vi "Cast IOLink Data.vi"(11 "System State In":map{string, dbl}(c390)) -> (3 "System State Out":map{string, dbl}(c390))   [LabVIEW 2024, in "Hardware Controller.lvlib"]
uses:
  Hardware Controller.lvlib
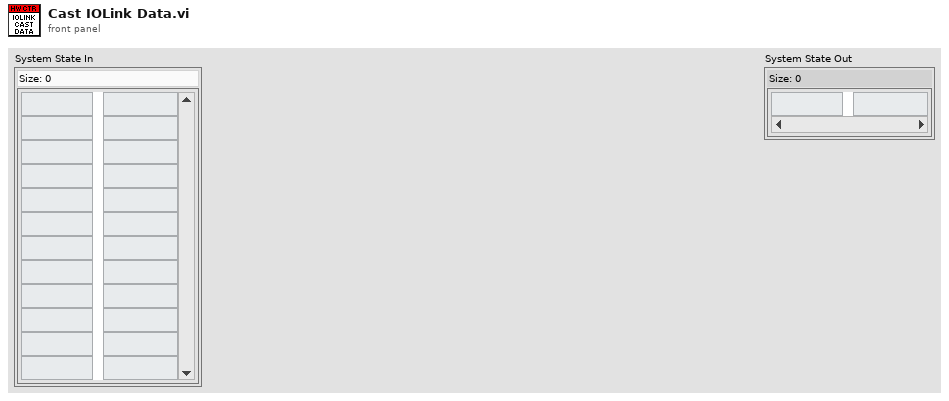
[diagram p1: front panel]
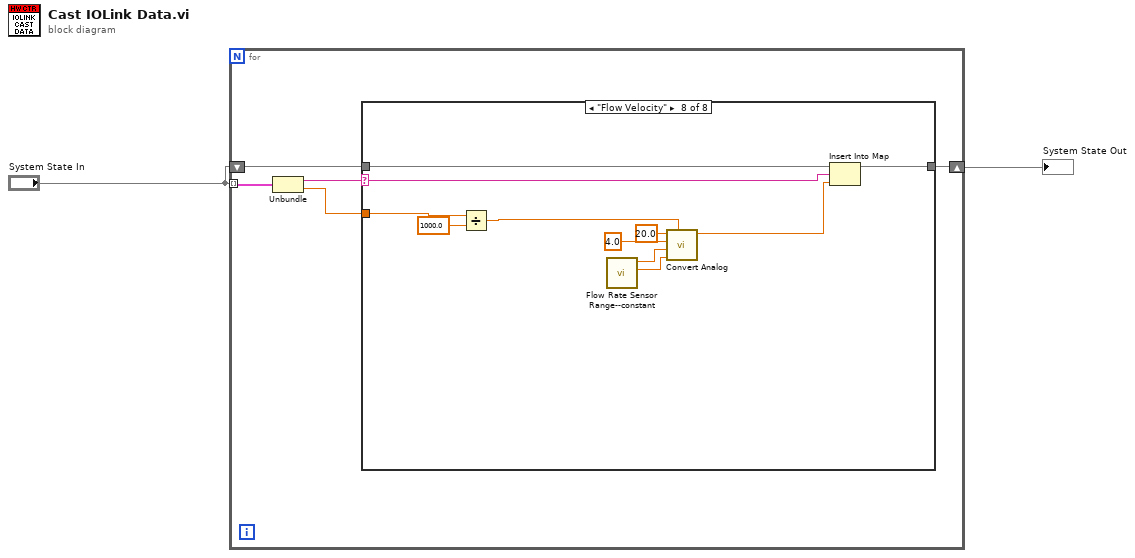
[diagram p0: block diagram]
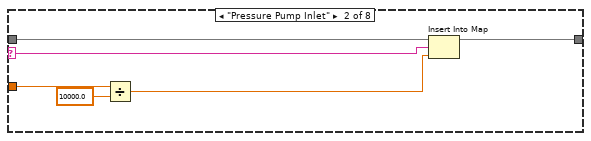
[diagram p3: hidden frame]
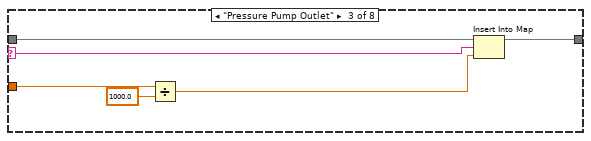
[diagram p4: hidden frame]
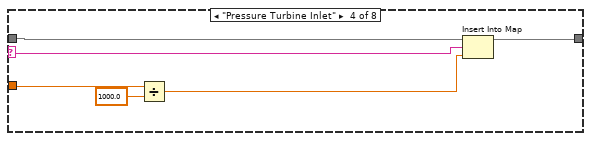
[diagram p5: hidden frame]
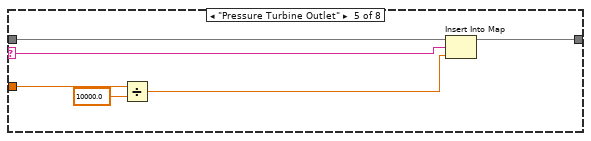
[diagram p6: hidden frame]
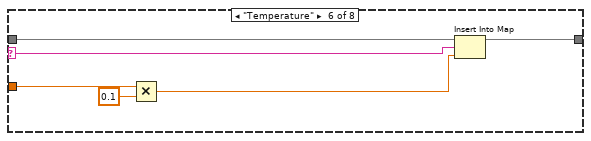
[diagram p7: hidden frame]
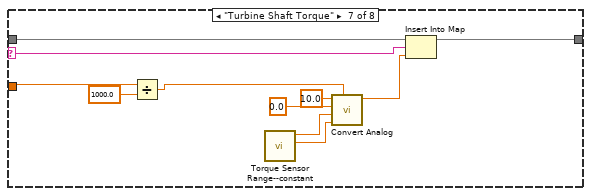
[diagram p8: hidden frame]
diagram:
  n1 = for {
    tunnel: "System State In" -> [w7] mode=indexing
    shift-right: [w3] -> w2
    shift-left: "System State In" -> [w6]
    n2 = Unbundle(w7) -> (w5:string, w4:dbl)
    n3 = case shown="\"Flow Velocity\"" w5 {
      selector: w5 -> [_ w10 w17 w22 w29 w35 w43 w56]
      tunnel: w6 -> [w8 w11 w16 w23 w30 w36 w44 w57]
      tunnel: w4 -> [_ w14 w18 w21 w28 w34 w40 w52]
      tunnel: [w8 w12 w15 w24 w27 w33 w45 w55] -> w3
      frame Default {
      }
      frame "Pressure Pump Inlet" {
        n4 = Divide(x=w14, y=10000.0) -> (x/y=w9:dbl)
        n5 = Insert Into Map(map in=w11, key=w10, value=w9) -> (map out=w12:map{string, dbl})  [unwired: 2 out]
      }
      frame "Pressure Pump Outlet" {
        n6 = Divide(x=w18, y=1000.0) -> (x/y=w19:dbl)
        n7 = Insert Into Map(map in=w16, key=w17, value=w19) -> (map out=w15:map{string, dbl})  [unwired: 2 out]
      }
      frame "Pressure Turbine Inlet" {
        n8 = Divide(x=w21, y=1000.0) -> (x/y=w25:dbl)
        n9 = Insert Into Map(map in=w23, key=w22, value=w25) -> (map out=w24:map{string, dbl})  [unwired: 2 out]
      }
      frame "Pressure Turbine Outlet" {
        n10 = Divide(x=w28, y=10000.0) -> (x/y=w31:dbl)
        n11 = Insert Into Map(map in=w30, key=w29, value=w31) -> (map out=w27:map{string, dbl})  [unwired: 2 out]
      }
      frame "Temperature" {
        n12 = Multiply(x=w34, y=0.1) -> (x*y=w37:dbl)
        n13 = Insert Into Map(map in=w36, key=w35, value=w37) -> (map out=w33:map{string, dbl})  [unwired: 2 out]
      }
      frame "Turbine Shaft Torque" {
        n14 = Divide(x=w40, y=1000.0) -> (x/y=w39:dbl)
        n15 = call "Torque Sensor Range--constant.vi"() -> ("Min"=w46:dbl, "Max"=w47:dbl)  [unwired: 10 in]
        n16 = call "Convert Analog.vi"("Input Value"=w39, "Sensor Min"=w46, "Sensor Max"=w47, "Signal Min"=0.0, "Signal Max"=10.0) -> ("result"=w42:dbl)  [unwired: 6 in]
        n17 = Insert Into Map(map in=w44, key=w43, value=w42) -> (map out=w45:map{string, dbl})  [unwired: 2 out]
      }
      frame "Flow Velocity" {
        n18 = Divide(x=w52, y=1000.0) -> (x/y=w50:dbl)
        n19 = call "Flow Rate Sensor Range--constant.vi"() -> ("Min"=w53:dbl, "Max"=w54:dbl)  [unwired: 10 in]
        n20 = call "Convert Analog.vi"("Input Value"=w50, "Sensor Min"=w53, "Sensor Max"=w54, "Signal Min"=4.0, "Signal Max"=20.0) -> ("result"=w60:dbl)  [unwired: 6 in]
        n21 = Insert Into Map(map in=w57, key=w56, value=w60) -> (map out=w55:map{string, dbl})  [unwired: 2 out]
      }
    }
  }
  "System State Out" <- w2
